vi "MyG#G3SubTempl_GetClassAttributesToModify.vi"(0 "reference in":refnum<class "MyG#G3SubTempl.lvclass">, 3 "timeout in ms (-1)":i32=-1, 5 "error in (no error)":errorcluster) -> (14 "reference out":refnum<class "MyG#G3SubTempl.lvclass">, 15 "class attributes ref":T3, 16 "class attributes":T1, 17 "timeout":bool, 18 "created new":bool, 19 "error out":errorcluster)   [LabVIEW 2017, in "MyG#G3SubTempl.lvclass"]
doc: "This VI returns the attributes associated with this class or subclass object reference and places a lock on the object.\n\nIf the object is currently locked for modification by another method, 'Timeout' specifies how long the VI should wait to receive access to the object. The default value waits until the object becomes available.\n\nYou must use this class SetModifiedAttributes VI to set the object's data and release the lock."
uses:
  MyG#G3SubTempl.lvclass
  C:/Projects/GsharpGIT/G# Framework/examples/AddQ/G#/CreateDestroy/MyG#G3Templ_class/MyG#G3Templ.lvclass
  ClassAttributesRef.ctl
  protected/ClassAttributes.ctl
  MyG#G3Templ_class/protected/ClassAttributes.ctl
  MyG#G3SubTempl.lvclass/MyG#G3SubTempl.ctl
  MyG#G3Templ_class/MyG#G3Templ.lvclass
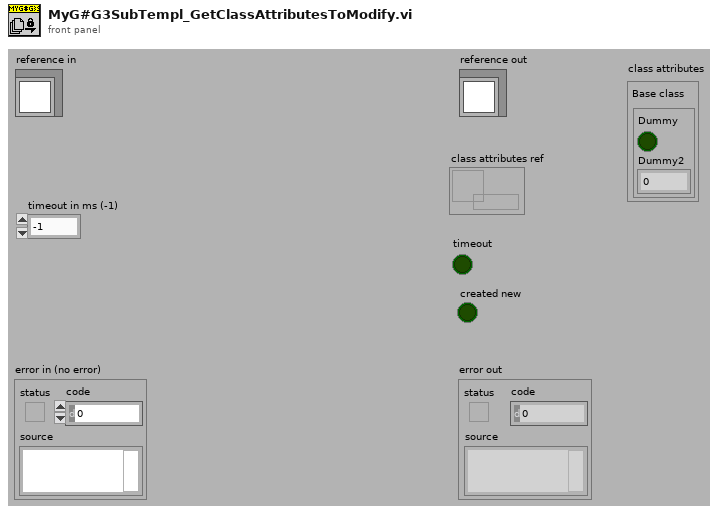
[diagram p1: front panel]
types:
  T1 = typedef "MyG#G3SubTempl.lvclass/ClassAttributes.ctl" = cluster{"Base class":T2}
  T2 = typedef "MyG#G3Templ.lvclass/ClassAttributes.ctl" = cluster{"Dummy":bool, "Dummy2":dbl}
  T3 = typedef "MyG#G3SubTempl.lvclass/ClassAttributesRef.ctl" = refnum<data-value>
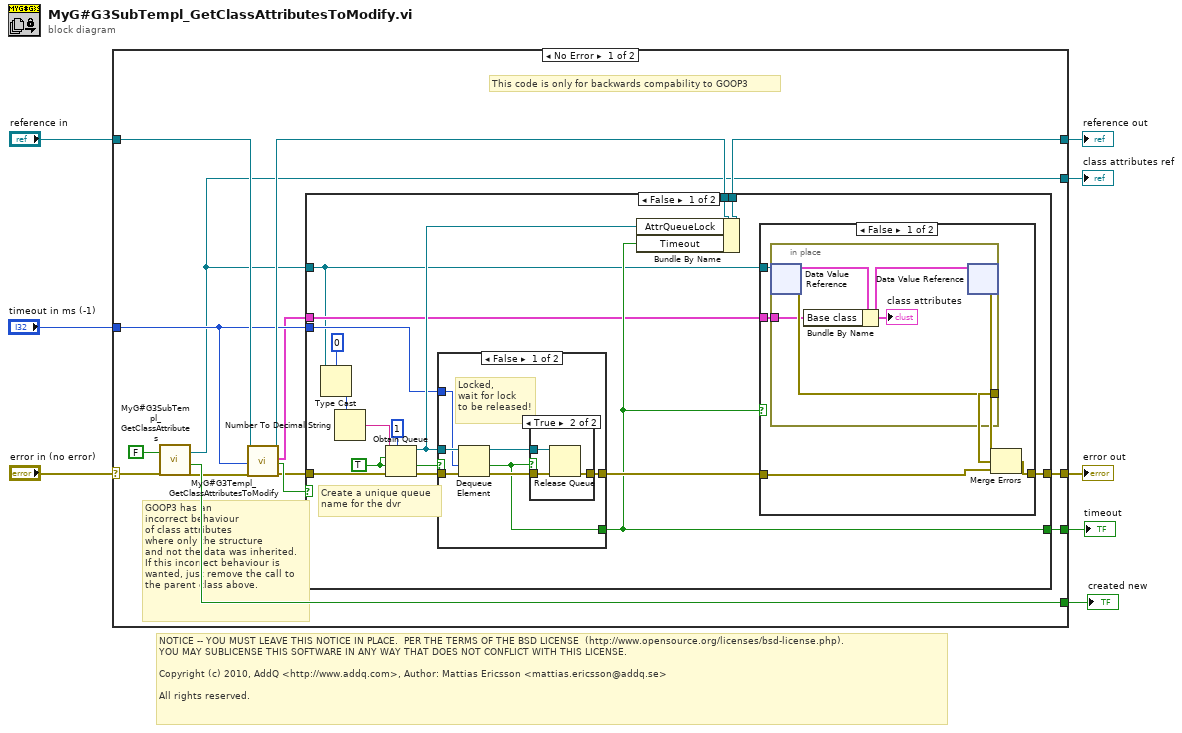
[diagram p0: block diagram]
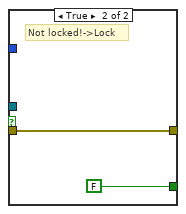
[diagram p3: hidden frame]
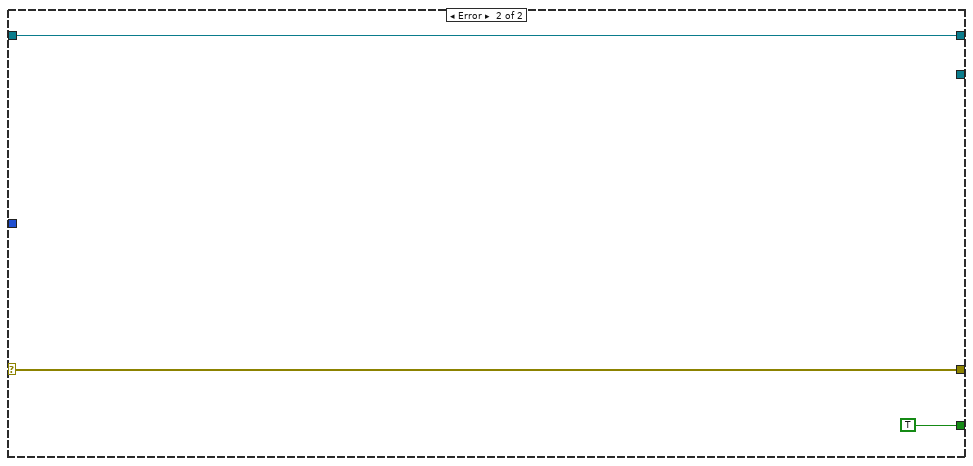
[diagram p6: hidden frame]
diagram:
  # "NOTICE -- YOU MUST LEAVE THIS NOTICE IN PLACE.  PER THE TERMS OF THE BSD LICENSE  (http://www.opensource.org/licenses/bsd-license.php).\nYOU MAY SUBLICENSE THIS SOFTWARE IN ANY WAY THAT DOES NOT CONFLICT WITH THIS LICENSE.\n\nCopyright (c) 2010, AddQ <http://www.addq.com>, Author: Mattias Ericsson <mattias.ericsson@addq.se>\n\nAll rights reserved."
  n1 = case shown="No Error" "error in (no error)" {
    selector: "error in (no error)" -> [w9 w69]
    tunnel: [w22 w69] -> w7
    tunnel: [w17 w68] -> w5
    tunnel: "reference in" -> [w20 w68]
    tunnel: [w13 _] -> w4
    tunnel: "timeout in ms (-1)" -> [w18 _]
    tunnel: [w16 TRUE ("status")] -> w2
    tunnel: [w11 _] -> w1
    frame No Error {
      # "GOOP3 has an\nincorrect behaviour\nof class attributes\nwhere only the structure\nand not the data was inherited.\nIf this incorrect behaviour is\nwanted, just remove the call to\nthe parent class above."
      # "This code is only for backwards compability to GOOP3"
      n2 = call "MyG#G3SubTempl_GetClassAttributes.vi"("return data"=FALSE, "error in (no error)"=w9) -> ("class attributes ref"=w13:T3, "created new"=w11:bool, "error out"=w10:errorcluster)  [unwired: 13 in, 2 out]
      n3 = call "MyG#G3Templ_GetClassAttributesToModify.vi"("reference in"=w20, "timeout in ms (-1)"=w18, "error in (no error)"=w10) -> ("reference out"=w19:refnum<class "MyG#G3SubTempl.lvclass">, "class attributes"=w15:T2, "timeout"=w14:bool, "error out"=w12:errorcluster)  [unwired: 11 in, 2 out]
      n4 = case shown="False" w14 {
        selector: w14 -> [_ w65]
        tunnel: [w39 w64] -> w22
        tunnel: w12 -> [w31 w64]
        tunnel: w19 -> [w28 w66]
        tunnel: w18 -> [w27 _]
        tunnel: [w26 w66] -> w17
        tunnel: [w25 w65] -> w16
        tunnel: w15 -> [w24 _]
        tunnel: w13 -> [w23 _]
        frame False {
          w37 = TRUE ("create if not found? (T)")
          # "Create a unique queue\nname for the dvr"
          n5 = Type Cast(type=u32 0, x=w23) -> (*(type *) &x=w30:u32)
          n6 = Number To Decimal String(number=w30) -> (decimal integer string=w38:string)  [unwired: 1 in]
          n7 = Obtain Queue(max queue size (-1, unlimited)=1, name (unnamed)=w38, element data type=w37, create if not found? (T)=w37, error in (no error)=w31) -> (queue out=w32:refnum<queue>, created new?=w34:bool, error out=w35:errorcluster)
          n8 = case shown="False" w34 {
            tunnel: w35 -> [w44 w51]
            tunnel: [w43 w51] -> w33
            tunnel: w32 -> [w46 _]
            tunnel: w27 -> [w45 _]
            tunnel: [w40 FALSE ("status")] -> w25
            frame False {
              # "Locked,\nwait for lock\nto be released!"
              n9 = Dequeue Element(queue=w46, timeout in ms (-1)=w45, error in (no error)=w44) -> (queue out=w41:refnum<queue>, timed out?=w40:bool, error out=w42:errorcluster)  [unwired: 1 out]
              n10 = case shown="True" w40 {
                tunnel: [w47 w50] -> w43
                tunnel: w42 -> [w47 w49]
                tunnel: w41 -> [_ w48]
                frame False {
                }
                frame True {
                  n11 = Release Queue(queue=w48, error in (no error)=w49) -> (error out=w50:errorcluster)  [unwired: 1 in, 2 out]
                }
              }
            }
            frame True {
              # "Not locked!->Lock"
            }
          }
          n12 = Bundle By Name(cluster=w28, "AttrQueueLock"=w32, "Timeout"=w25) -> (w26:refnum<class "MyG#G3SubTempl.lvclass">)
          n13 = case shown="False" w25 {
            tunnel: w23 -> [w58 _]
            tunnel: w33 -> [w57 w63]
            tunnel: [w54 w63] -> w39
            tunnel: w24 -> [w53 _]
            frame False {
              n14 = in-place {
                in-place-border: [w60] -> w56
                in-place-border: w53 -> [w59]
                n15 = in-place-dvr #1(w58) -> (w62:T1, w60:errorcluster)
                n16 = Bundle By Name(cluster=w62, "Base class"=w59) -> (w61:T1)
                "class attributes" <- w61
                n17 = in-place-dvr #1(w61) -> (w55:errorcluster)  [unwired: 1 out]
              }
              n18 = Merge Errors(w55, w56, w57) -> (w54:errorcluster)
            }
            frame True {
              # "Timeout"
            }
          }
        }
        frame True {
        }
      }
    }
    frame Error {
    }
  }
  "error out" <- w7
  "reference out" <- w5
  "class attributes ref" <- w4
  "timeout" <- w2
  "created new" <- w1
